vi "DAQOutputInitialize.vi"(8 "error in (no error)":errorcluster, 11 "Data Cluster in":T1) -> (0 "error out":errorcluster, 2 "error?":bool, 3 "Data Cluster out":T1)   [LabVIEW 2026, in "Control.lvlib"]
uses:
  Control.lvlib
  Acquisition/Hardware Configuration.ctl
  controls/Durability Test Conditions.ctl
  <vilib>/DAQmx/create/channels.llb/DAQmx Create Channel (DO-Digital Output).vi
  Acquisition/Acquisition.lvlib
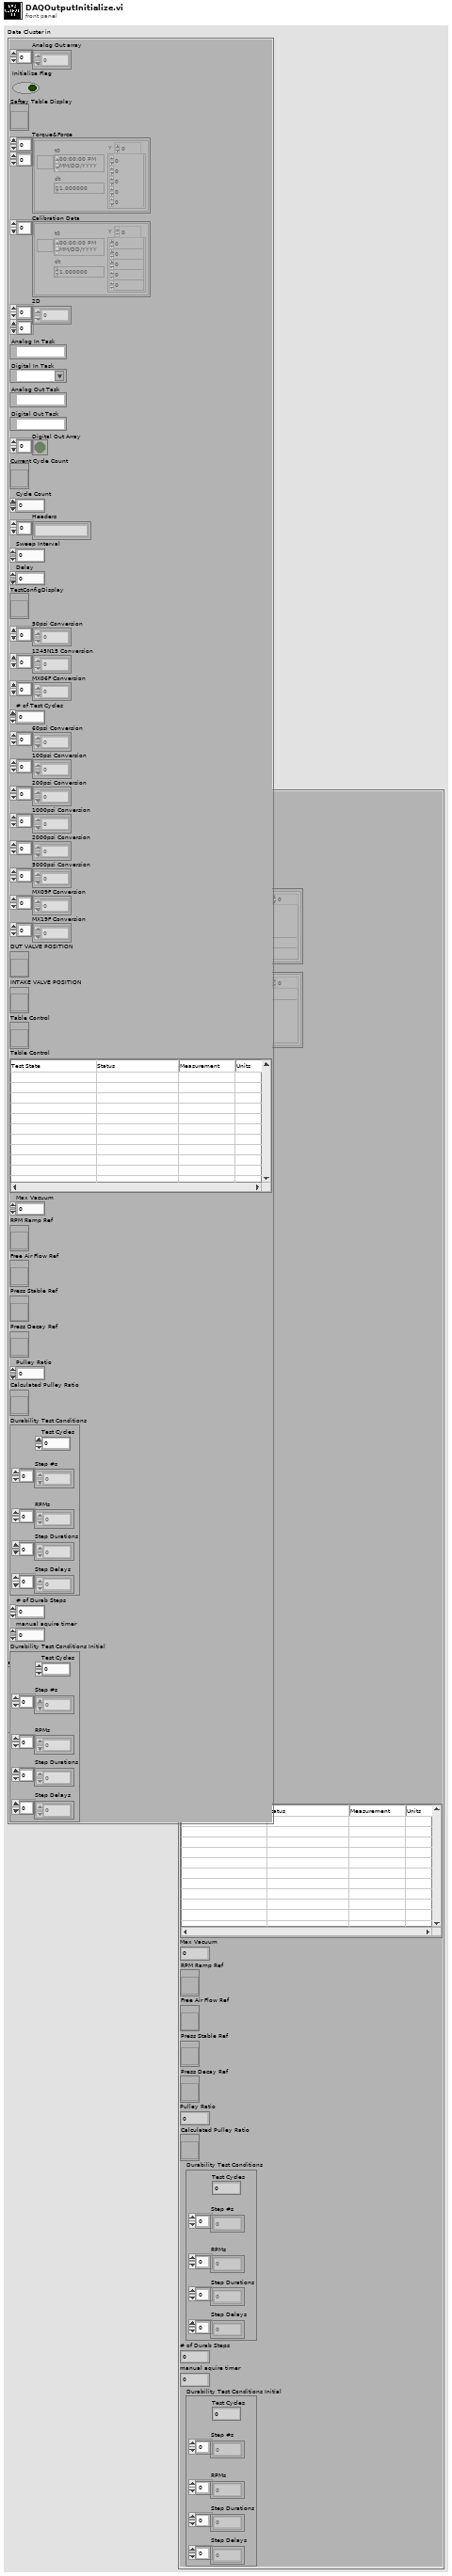
[diagram p1: front panel]
types:
  T1 = typedef "Acquisition.lvlib/Hardware Configuration.ctl" = cluster{"Analog Out array":dbl[], "Initialize Flag":bool, "Saftey Table Display":refnum<vi>, "Torque&Force":waveform(dbl)[][], "Calibration Data":waveform(dbl)[], "2D":dbl[][], "Analog In Task":refnum<k21>, "Digital In Task":refnum<k21>, "Analog Out Task":refnum<k21>, "Digital Out Task":refnum<k21>, "Digital Out Array":bool[], "Current Cycle Count":refnum<vi>, "Cycle Count":u64, "Headers":string[], "Sweep Interval":u64, "Delay":u64, "TestConfigDisplay":refnum<vi>, "50psi Conversion":dbl[], "1245N15 Conversion":dbl[], "MX06F Conversion":dbl[], "# of Test Cycles":u64, "60psi Conversion":dbl[], "100psi Conversion":dbl[], "200psi Conversion":dbl[], "1000psi Conversion":dbl[], "2000psi Conversion":dbl[], "5000psi Conversion":dbl[], "MX09F Conversion":dbl[], "MX19F Conversion":dbl[], "DUT VALVE POSITION":refnum<vi>, "INTAKE VALVE POSITION":refnum<vi>, "Table Control":refnum<vi>, "Table Control":string[][], "Max Vacuum":dbl, "RPM Ramp Ref":refnum<vi>, "Free Air Flow Ref":refnum<vi>, "Press Stable Ref":refnum<vi>, "Press Decay Ref":refnum<vi>, "Pulley Ratio":dbl, "Calculated Pulley Ratio":refnum<vi>, "Durability Test Conditions":T2, "# of Durab Steps":dbl, "manual aquire timer":dbl, "Durability Test Conditions Initial":T2}
  T2 = typedef "Durability Test Conditions.ctl" = cluster{"Step #s":dbl[], "RPMs":dbl[], "Step Durations":dbl[], "Step Delays":dbl[], "Test Cycles":dbl}
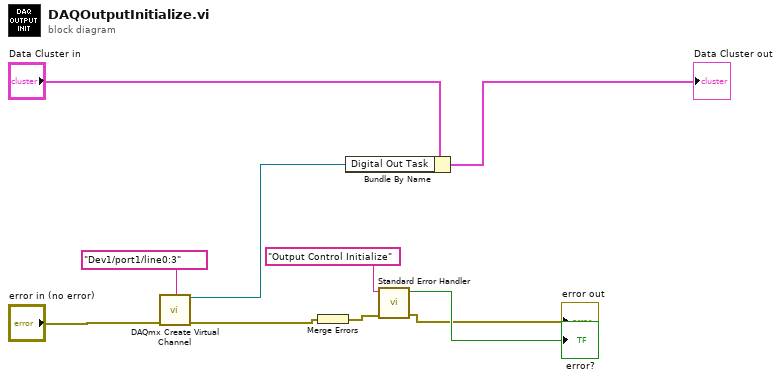
[diagram p0: block diagram]
diagram:
  n1 = call-poly <vilib>:"DAQmx Create Virtual Channel.vi"("lines"=tag "Dev1/port1/line0:3", "error in"="error in (no error)") -> ("task out"=w10:refnum<k21>, "error out"=w7:errorcluster)  [unwired: 12 in]
  n2 = Merge Errors(w7) -> (w4:errorcluster)
  n3 = Bundle By Name(cluster="Data Cluster in", "Digital Out Task"=w10) -> (→"Data Cluster out":T1)
  n4 = call "Standard Error Handler.vi"("error in (no error)"=w4, "source"="Output Control Initialize") -> ("error out"=→"error out":errorcluster, "error?"=→"error?":bool)  [unwired: 8 in]
